vi "read_bin1.vi"(4 "error in":errorcluster, 5 "Array":waveform(i16)[](array[waveform]), 7 "Path":path=path "79-2009_11_26-12_33_00.dat") -> (0 "error out":errorcluster, 1 "Waveform Graph":waveform(i16)[](graph), 3 "new file path":path=path "U:/Andrew/Andrew_STEND/РПГНы Тюмени/SKIL2_78/LV_work/Processing/79-2009_11_26-12_33_00.dat")   [LabVIEW 2010]
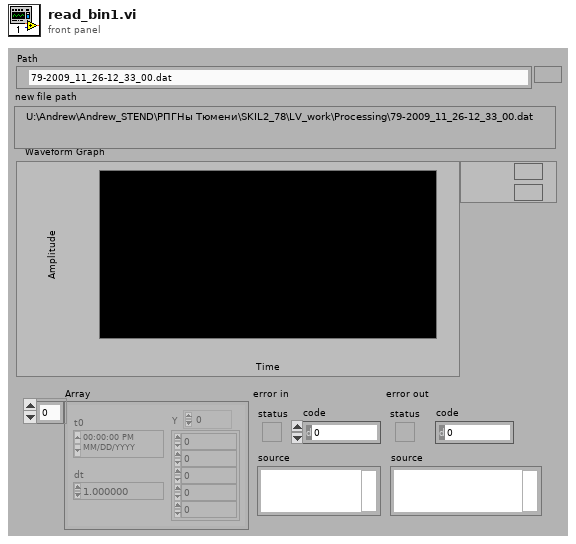
[diagram p1: front panel]
types:
  T1 = enum32{"existing file", "new file", "new or existing file", "existing dir", "new dir", "new or existing dir", "existing file (use LLBs)", "new file (use LLBs)", "new or existing file (use LLBs)", "new or existing file or directory (use LLBs)"}
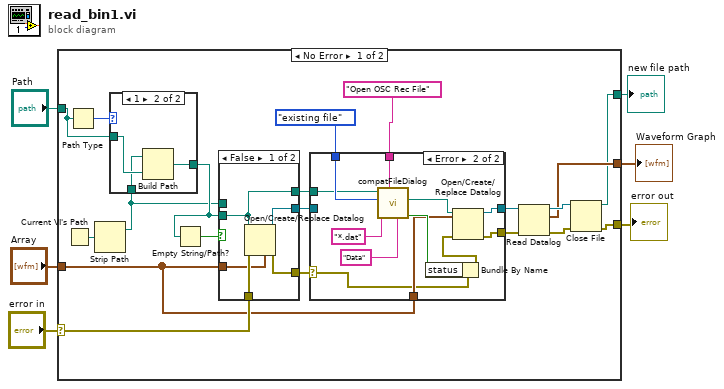
[diagram p0: block diagram]
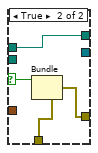
[diagram p2: hidden frame]
diagram:
  n1 = case shown="No Error" "error in" {
    selector: "error in" -> [w16 w56]
    tunnel: [w24 w56] -> w6
    tunnel: "Array" -> [w15 w55]
    tunnel: [w19 w55] -> w4
    tunnel: [w12 w54] -> w2
    tunnel: "Path" -> [w17 w54]
    frame No Error {
      n2 = Current VI's Path() -> (path=w11:path)
      n3 = Path Type(1:w17) -> (0:w18:i16)
      n4 = Strip Path(path=w11) -> (stripped path=w7:path)  [unwired: 1 out]
      n5 = case shown="1" w18 {
        tunnel: w17 -> [w50 w53]
        tunnel: [w50 w52] -> w9
        tunnel: w7 -> [_ w51]
        frame 0, Default {
        }
        frame 1 {
          n6 = Build Path(base path=w51, name or relative path=w53) -> (appended path=w52:path)
        }
      }
      n7 = Empty String/Path?(string/path=w9) -> (empty?=w10:bool)
      n8 = case shown="False" w10 {
        selector: w10 -> [_ w34]
        tunnel: w9 -> [w27 _]
        tunnel: w16 -> [w31 w35]
        tunnel: w15 -> [w30 _]
        tunnel: [w29 w33] -> w14
        tunnel: [w28 _] -> w13
        tunnel: [w27 w32] -> w8
        tunnel: w7 -> [_ w32]
        frame False {
          n9 = Open/Create/Replace Datalog(5:w30, 8:w31, 11:w27) -> (0:w29:errorcluster, 3:w28:refnum<k1>)  [unwired: 3 in, 1 out]
        }
        frame True {
          n10 = Bundle(cluster=w35, "status"=w34) -> (w33:errorcluster)  [unwired: 2 in]
        }
      }
      n11 = case shown="Error" w14 {
        selector: w14 -> [w36 w41]
        tunnel: [w36 w49] -> w23
        tunnel: [w37 w48] -> w22
        tunnel: T1."existing file" ("select mode (2)") -> [_ w47]
        tunnel: "Open OSC Rec File" ("prompt") -> [_ w46]
        tunnel: w15 -> [_ w42]
        tunnel: w13 -> [w37 _]
        tunnel: w8 -> [_ w38]
        frame No Error {
        }
        frame Error {
          n12 = call <vilib>:"compatFileDialog.vi"("pattern label"="Data", "prompt"=w46, "pattern"="*.dat", "select mode (2)"=w47, "start path"=w38) -> ("cancelled"=w45:bool, "path"=w43:path)  [unwired: 4 in, 1 out]
          n13 = Bundle By Name(cluster=w41, "status"=w45) -> (w44:errorcluster)
          n14 = Open/Create/Replace Datalog(5:w42, 8:w44, 11:w43) -> (0:w49:errorcluster, 3:w48:refnum<k1>)  [unwired: 3 in, 1 out]
        }
      }
      n15 = Read Datalog(4:w23, 7:w22) -> (0:w25:errorcluster, 2:w19:waveform(i16)[], 3:w26:refnum<k1>)  [unwired: 1 in]
      n16 = Close File(refnum=w26, error in=w25) -> (path=w12:path, error out=w24:errorcluster)
    }
    frame Error {
    }
  }
  "error out" <- w6
  "Waveform Graph" <- w4
  "new file path" <- w2
